vi "ep_Check Speed Nameplate for Single Motor.vi"(8 "error in (no error)":errorcluster, 9 "full load speed [RPM]":dbl, 10 "synchronous speed [RPM]":dbl, 11 "nominal frequency":enum16{"50 Hz", "60 Hz"}(ring)) -> (0 "error out":errorcluster)   [LabVIEW 2014, in "NI_EP_Motor Monitoring.lvlib"]
uses:
  <vilib>/addons/Electrical Power/Motor Monitoring/NI_EP_Motor Monitoring.lvlib
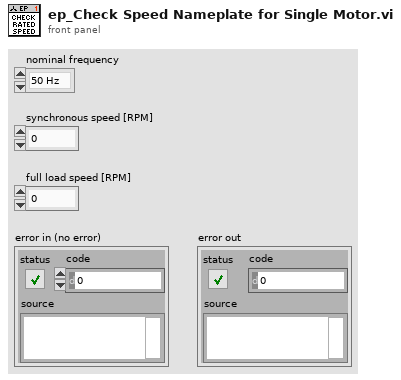
[diagram p1: front panel]
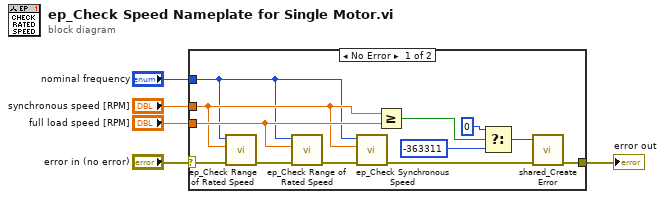
[diagram p0: block diagram]
diagram:
  n1 = case shown="No Error" "error in (no error)" {
    selector: "error in (no error)" -> [w13 w18]
    tunnel: "nominal frequency" -> [w7 _]
    tunnel: "full load speed [RPM]" -> [w11 _]
    tunnel: "synchronous speed [RPM]" -> [w8 _]
    tunnel: [w6 w18] -> w1
    frame No Error {
      n2 = call <vilib>:"ep_Check Range of Rated Speed.vi"("error in (no error)"=w13, "speed [RPM]"=w8, "nominal frequency"=w7) -> ("error out"=w12:errorcluster)  [unwired: 8 in]
      n3 = call <vilib>:"ep_Check Range of Rated Speed.vi"("error in (no error)"=w12, "speed [RPM]"=w11, "nominal frequency"=w7) -> ("error out"=w10:errorcluster)  [unwired: 8 in]
      n4 = call <vilib>:"ep_Check Synchronous Speed.vi"("error in (no error)"=w10, "synchronous speed [RPM]"=w8, "nominal frequency"=w7) -> ("error out"=w9:errorcluster)  [unwired: 8 in]
      n5 = Greater Or Equal?(x=w8, y=w11) -> (x >= y?=w17:bool)
      n6 = Select(t=0 ("y"), s=w17, f=-363311 ("y")) -> (s? t:f=w14:i32)
      n7 = call <vilib>:"shared_Create Error.vi"("error in (no error)"=w9, "error code (0)"=w14) -> ("error out"=w6:errorcluster)  [unwired: 9 in]
    }
    frame Error {
    }
  }
  "error out" <- w1
